vi "Worker List UI.vi"() -> ()   [LabVIEW 2020, in "FlexBlocks.lvlib"]
uses:
  FlexBlocks.lvlib
  UI State.ctl
panel:
  out "Icon":picture
  in  "New Variant":bool
  in  "Enable Variants":bool
  in  "Open Worker":bool
  in  "Values":string(tree)
  in  "New Worker":bool
  in  "Variant":i32(listbox)
  in  "Worker Search":string
  in  "Clear Search":bool
  out "Worker Name":string
  in  "Workers":i32(listbox)
  # "No variants for the selected worker"
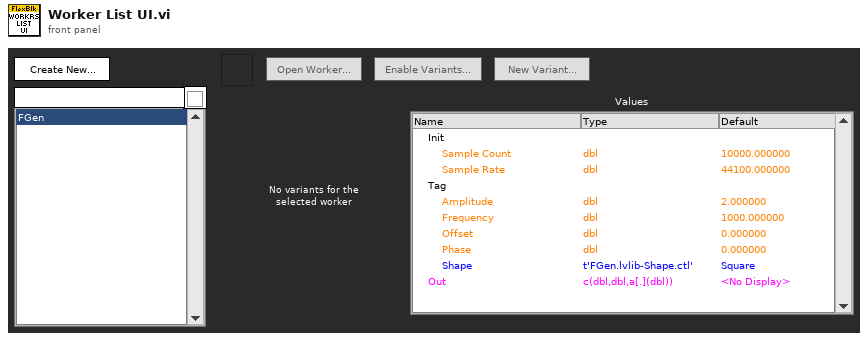
[diagram p1: front panel]
types:
  T1 = typedef "FlexBlocks.lvlib/UI State.ctl" = enum16{"Init", "Load", "Ready", "Run", "Close"}
  T2 = enum32{"Invalid", "Standard", "Closed", "Hidden", "Minimized", "Maximized"}
  T3 = enum8{"Enabled", "Disabled", "Disabled and Grayed Out"}
  T4 = typedef "imagedata.ctl" = cluster{"image type":i32, "image depth":i32, "image":u8[], "mask":u8[], "colors":u32[], "Rectangle":cluster{"left":i16, "top":i16, "right":i16, "bottom":i16}}
  T5 = typedef "FlexBlocks.lvlib/Special Terminal Indices.ctl" = cluster{"Action":i32, "Init":i32, "Tag":i32, "State in":i32, "State out":i32, "Error":i32}
  T6 = typedef "FlexBlocks.lvlib/Type Descriptor.ctl" = cluster{"Name":string, "Direction":T7, "Default":variant, "Min":variant, "Max":variant, "Step":variant, "Value Mode":T8, "Required":bool, "Connpane Index":i32, "Special Terminal":T9, "Color":u32, "Channel Path":path, "Options":string[], "Type String":string, "Sort":i32}
  T7 = typedef "FlexBlocks.lvlib/Terminal Direction.ctl" = enum16{"Sink", "Source"}
  T8 = typedef "FlexBlocks.lvlib/Value Mode.ctl" = enum16{"Normal", "Range", "Select"}
  T9 = typedef "FlexBlocks.lvlib/Special Terminal.ctl" = enum16{"None", "Action", "Init", "Tag", "State in", "State out", "Error"}
  T10 = typedef "eventvkey.ctl" = enum16{"ASCII", "Enter", "Return", "Shift", "Ctrl", "Alt", "Cmd", "Opt", "Caps", "NumLock", "Clear", "Break", "Up", "Down", "Left", "Right", "Insert", "Delete", "Home", "End", "PageUp", "PageDown", "Escape", "Help", "Pause", "ScrollLock", "F1", "F2", "F3", "F4", "F5", "F6", "F7", "F8", "F9", "F10", "F11", "F12", "F13", "F14", "F15", "F16", "F17", "F18", "F19", "F20", "F21", "F22", "F23", "F24", "Play", "VolumeUp", "VolumeDown", "Mute", "Two Byte Char"}
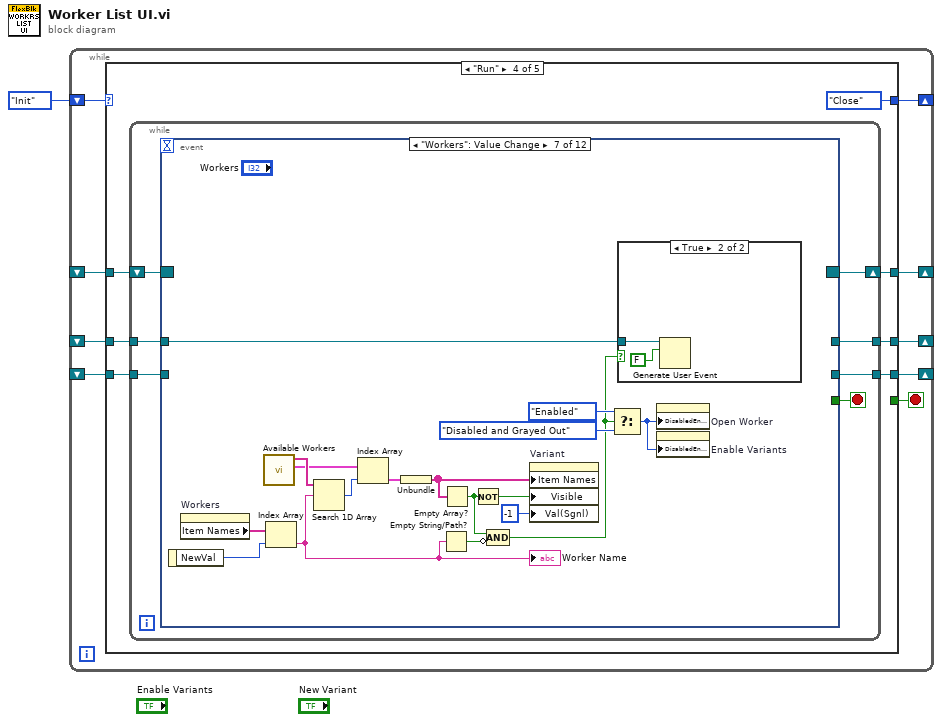
[diagram p0: block diagram]
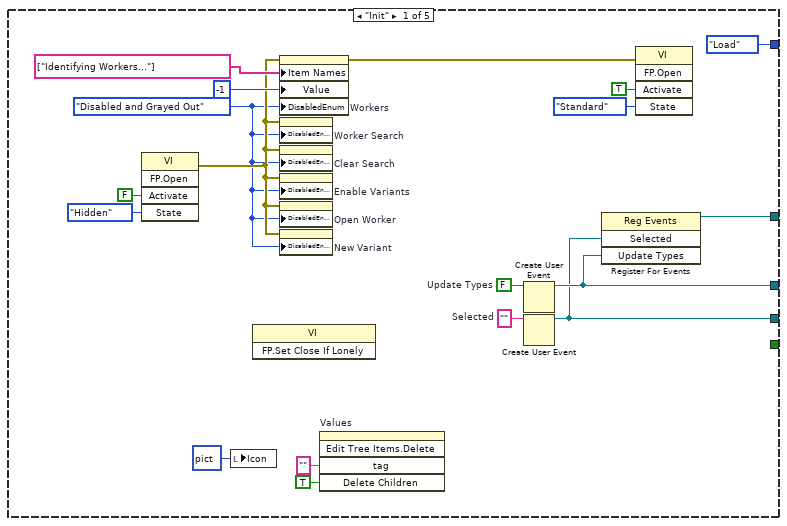
[diagram p2: hidden frame]
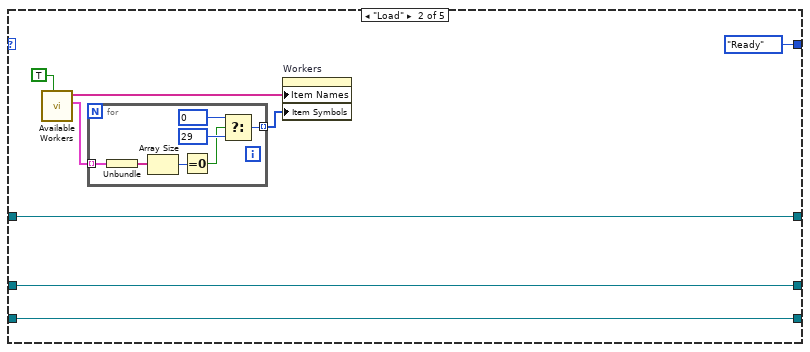
[diagram p3: hidden frame]
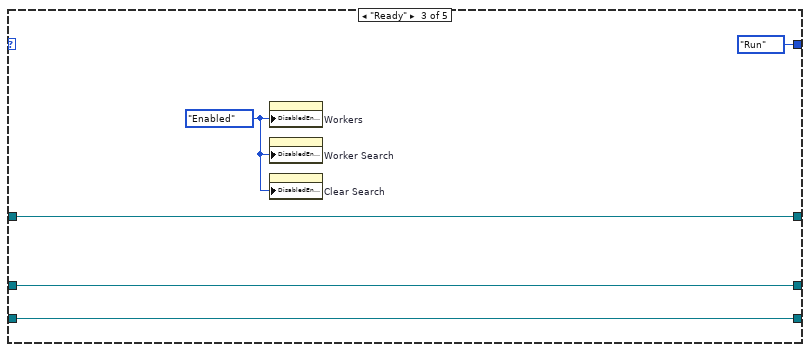
[diagram p4: hidden frame]
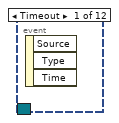
[diagram p5: hidden frame]
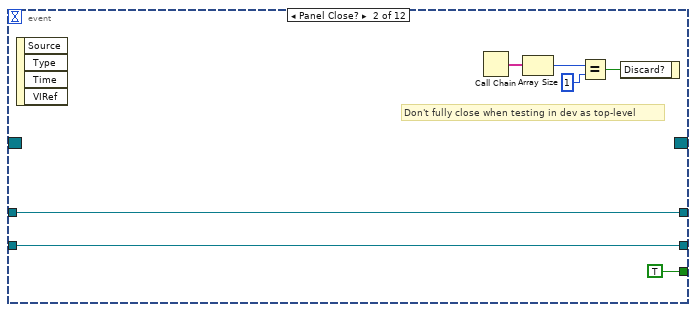
[diagram p6: hidden frame]
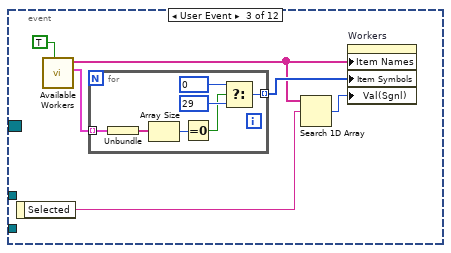
[diagram p7: hidden frame]
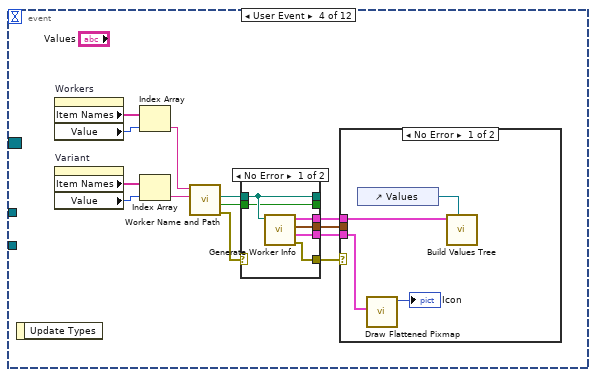
[diagram p8: hidden frame]
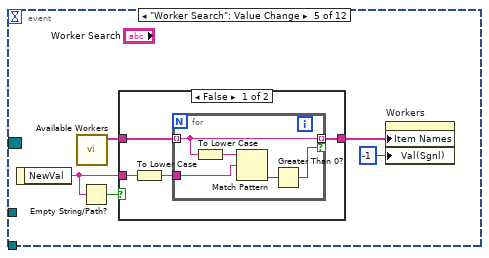
[diagram p11: hidden frame]
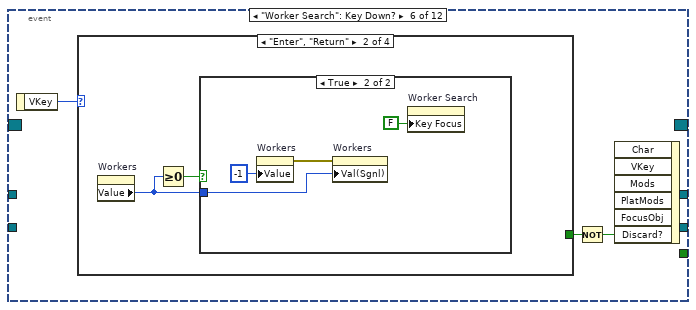
[diagram p13: hidden frame]
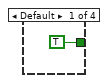
[diagram p14: hidden frame]
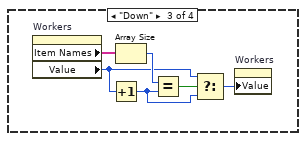
[diagram p16: hidden frame]
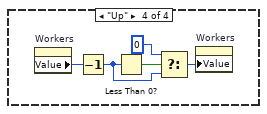
[diagram p17: hidden frame]
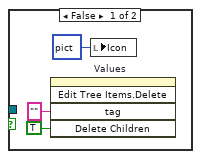
[diagram p18: hidden frame]
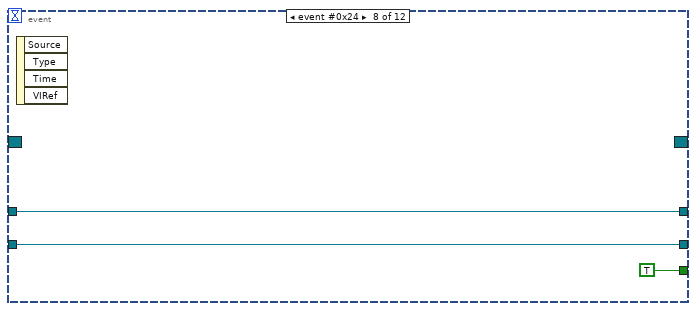
[diagram p19: hidden frame]
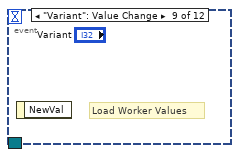
[diagram p20: hidden frame]
diagram:
  n1 = while {
    shift-right: [w9] -> _
    shift-left: UI_State."Init" ("UI State") -> [w10]
    shift-right: [w7] -> _
    shift-left: _ -> [w5]
    shift-right: [w6] -> _
    shift-left: _ -> [w4]
    shift-right: [w3] -> _
    shift-left: _ -> [w2]
    stop <- w8 stop-if-true
    n2 = case shown="\"Run\"" w10 {
      selector: w10 -> [_ _ _ _ w200]
      tunnel: [UI_State."Load" ("UI State") UI_State."Ready" ("UI State") UI_State."Run" ("UI State") UI_State."Close" ("UI State") w200] -> w9
      tunnel: [_ _ _ _ TRUE] -> w8
      tunnel: [w21 w31 w46 w52 refnum<event-registration> refnum ("Event Registration Refnum")] -> w7
      tunnel: [w14 w30 w45 w51 refnum<user-event> refnum ("Selected")] -> w6
      tunnel: w5 -> [_ w31 w46 w54 w197]
      tunnel: w4 -> [_ w30 w45 w53 w198]
      tunnel: [w15 w29 w44 w49 refnum<user-event> refnum ("Update Types")] -> w3
      tunnel: w2 -> [_ w29 w44 w50 w194]
      frame "Init" {
        w16 = FALSE  # Update Types
        w20 = ""  # Selected
        w18 = T3."Disabled and Grayed Out" ("Disabled")
        n3 = invoke class="VI" method="FP.Open"("Activate"=FALSE ("Activate?"), "State"=T2."Hidden") -> (error out=w19:errorcluster)  [unwired: 3 in, 4 out]
        n4 = local write "Icon"(picture data[5B] ("empty picture")) -> ()
        n5 = invoke class="VI" method="FP.Set Close If Lonely"() -> ()  [unwired: 3 in, 3 out]
        n6 = property on="Workers" class="LstBox (strict)"(error in=w19, "Item Names"=string[] ["Identifying Workers..."], "Value"=-1 ("Workers"), "DisabledEnum"=w18) -> (error out=w17:errorcluster)  [unwired: 1 in, 1 out]
        n7 = property on="Worker Search" class="Str"(error in=w19, "DisabledEnum"=w18) -> ()  [unwired: 1 in, 2 out]
        n8 = property on="Clear Search" class="Bool"(error in=w19, "DisabledEnum"=w18) -> ()  [unwired: 1 in, 2 out]
        n9 = property on="Enable Variants" class="Bool"(error in=w19, "DisabledEnum"=w18) -> ()  [unwired: 1 in, 2 out]
        n10 = property on="Open Worker" class="Bool"(error in=w19, "DisabledEnum"=w18) -> ()  [unwired: 1 in, 2 out]
        n11 = property on="New Variant" class="Bool"(error in=w19, "DisabledEnum"=w18) -> ()  [unwired: 1 in, 2 out]
        n12 = invoke on="Values" class="Tree (strict)" method="Edit Tree Items.Delete"("tag"="" ("Tag"), "Delete Children"=TRUE ("Delete Children?")) -> ()  [unwired: 3 in, 5 out]
        n13 = Create User Event(user event datatype=w16) -> (user event=w15:refnum<user-event>)  [unwired: 1 in, 1 out]
        n14 = Create User Event(user event datatype=w20) -> (user event=w14:refnum<user-event>)  [unwired: 1 in, 1 out]
        n15 = register-events(w14, w15) -> (reference out=w21:refnum<event-registration>)  [unwired: 2 in, 1 out]
        n16 = invoke class="VI" method="FP.Open"(error in=w17, "Activate"=TRUE ("Activate?"), "State"=T2."Standard") -> ()  [unwired: 2 in, 5 out]
      }
      frame "Load" {
        n17 = call "Available Workers.vi"("Refresh? (F)"=TRUE) -> ("Variants"=w33:cluster{"Variants":string[]}[], "Available Workers"=w34:string[])  [unwired: 9 in]
        n18 = for {
          tunnel: w33 -> [w41] mode=indexing
          tunnel: [w37] -> w32 mode=indexing
          n19 = Unbundle(w41) -> ("Variants"=w40:string[])
          n20 = Array Size(array=w40) -> (size(s)=w39:i32)
          n21 = Equal To 0?(x=w39) -> (x = 0?=w38:bool)
          n22 = Select(t=0, s=w38, f=29) -> (s? t:f=w37:i32)
        }
        n23 = property on="Workers" class="LstBox (strict)"("Item Names"=w34, "Item Symbols"=w32) -> ()  [unwired: 2 in, 2 out]
      }
      frame "Ready" {
        w47 = T3."Enabled" ("Disabled")
        n24 = property on="Workers" class="LstBox (strict)"("DisabledEnum"=w47) -> ()  [unwired: 2 in, 2 out]
        n25 = property on="Worker Search" class="Str"("DisabledEnum"=w47) -> ()  [unwired: 2 in, 2 out]
        n26 = property on="Clear Search" class="Bool"("DisabledEnum"=w47) -> ()  [unwired: 2 in, 2 out]
      }
      frame "Run" {
        n27 = while {
          shift-right: [w59] -> w52
          shift-left: w54 -> [w61]
          tunnel: w53 -> [w60]
          tunnel: [w58] -> w51
          tunnel: w50 -> [w57]
          tunnel: [w56] -> w49
          stop <- w62 stop-if-true
          n28 = event shown="[6] \"Workers\": Value Change" {
            selector: w61 -> [_ _ _ _ _ _ _ _ _ _ _ _]
            dyn-events: [_ _ _ _ _ _ _ _ _ _ _ _] -> w59
            timeout: _ -> [_ _ _ _ _ _ _ _ _ _ _ _]
            tunnel: [_ TRUE _ _ _ _ _ TRUE _ _ _ _] -> w62
            tunnel: w60 -> [_ w68 _ _ _ _ _ w167 _ _ w169 _]
            tunnel: [_ w68 _ _ _ _ _ w167 _ _ _ _] -> w58
            tunnel: w57 -> [_ w63 _ _ _ _ w144 w165 _ _ _ _]
            tunnel: [_ w63 _ _ _ _ _ w165 _ _ _ _] -> w56
            event Timeout {
              n29 = event-data() -> ()  [unwired: 1 in, 3 out]
            }
            event Panel Close? {
              # "Don't fully close when testing in dev as top-level"
              n30 = event-data() -> ()  [unwired: 1 in, 4 out]
              n31 = Call Chain() -> (call chain=w67:string[])
              n32 = Array Size(array=w67) -> (size(s)=w66:i32)
              n33 = Equal?(x=w66, y=1) -> (x = y?=w64:bool)
              n34 = event-data("Discard?"=w64) -> ()  [unwired: 1 in, 1 out]
            }
            event User Event {
              n35 = event-data() -> ("Selected"=w71:string)  [unwired: 1 in]
              n36 = call "Available Workers.vi"("Refresh? (F)"=TRUE) -> ("Variants"=w74:cluster{"Variants":string[]}[], "Available Workers"=w72:string[])  [unwired: 9 in]
              n37 = for {
                tunnel: w74 -> [w80] mode=indexing
                tunnel: [w76] -> w73 mode=indexing
                n38 = Unbundle(w80) -> ("Variants"=w79:string[])
                n39 = Array Size(array=w79) -> (size(s)=w78:i32)
                n40 = Equal To 0?(x=w78) -> (x = 0?=w77:bool)
                n41 = Select(t=0, s=w77, f=29) -> (s? t:f=w76:i32)
              }
              n42 = Search 1D Array(1D array=w72, element=w71) -> (index of element=w70:i32)  [unwired: 1 in]
              n43 = property on="Workers" class="LstBox (strict)"("Item Names"=w72, "Item Symbols"=w73, "Val(Sgnl)"=w70) -> ()  [unwired: 2 in, 2 out]
            }
            event User Event {
              n44 = event-data() -> ()  [unwired: 1 in, 1 out]
              n45 = property on="Workers" class="LstBox (strict)"() -> ("Item Names"=w92:string[], "Value"=w91:i32)  [unwired: 2 in, 2 out]
              n46 = property on="Variant" class="LstBox (strict)"() -> ("Item Names"=w89:string[], "Value"=w90:i32)  [unwired: 2 in, 2 out]
              n47 = Index Array(array=w92, index=w91) -> (element=w87:string)
              n48 = Index Array(array=w89, index=w90) -> (element=w88:string)
              n49 = call "Worker Name and Path.vi"("Variant"=w88, "Worker"=w87) -> ("error out"=w94:errorcluster, "Is Worker Variant"=w93:bool, "lvlib Path"=w95:path)  [unwired: 6 in, 1 out]
              n50 = case shown="No Error" w94 {
                selector: w94 -> [_ w106]
                tunnel: [w105 w106] -> w86
                tunnel: [w104 _] -> w85
                tunnel: [w103 _] -> w84
                tunnel: [w102 _] -> w83
                tunnel: w95 -> [w101 _]
                tunnel: [w101 _] -> _
                tunnel: w93 -> [w100 _]
                tunnel: [w100 _] -> _
                frame No Error {
                  n51 = call "Generate Worker Info.vi"("Worker lvlib"=w101) -> ("error out"=w105:errorcluster, "Icon"=w104:T4, "Special Terminals"=w103:T5, "Type Descriptors"=w102:T6[])  [unwired: 7 in]
                }
                frame Error {
                }
              }
              n52 = case shown="No Error" w86 {
                tunnel: w85 -> [w99 _]
                tunnel: w84 -> [_ _]
                tunnel: w83 -> [w97 _]
                frame No Error {
                  n53 = control-ref of="Values"() -> (w96:refnum<vi>)
                  n54 = call <vilib>:"Draw Flattened Pixmap.vi"("image data"=w99) -> ("new picture"=→"Icon":picture)  [unwired: 8 in]
                  n55 = call "Build Values Tree.vi"("Tree"=w96, "Types"=w97) -> ()  [unwired: 10 in]
                }
                frame Error {
                }
              }
            }
            event "Worker Search": Value Change {
              n56 = event-data() -> ("NewVal"=w110:string)  [unwired: 1 in]
              n57 = call "Available Workers.vi"() -> ("Available Workers"=w111:string[])  [unwired: 10 in, 1 out]
              n58 = Empty String/Path?(string/path=w110) -> (empty?=w109:bool)
              n59 = case shown="False" w109 {
                tunnel: w111 -> [w115 w121]
                tunnel: w110 -> [w114 _]
                tunnel: [w113 w121] -> w108
                frame False {
                  n60 = To Lower Case(string=w114) -> (all lower case string=w112:string)
                  n61 = for {
                    tunnel: w115 -> [w120] mode=indexing
                    tunnel: w112 -> [w119]
                    tunnel: [w120] -> w113 mode=indexing if=w117
                    n62 = To Lower Case(string=w120) -> (all lower case string=w116:string)
                    n63 = Match Pattern(string=w116, regular expression=w119) -> (offset past match=w118:i32)  [unwired: 1 in, 3 out]
                    n64 = Greater Than 0?(x=w118) -> (x > 0?=w117:bool)
                  }
                }
                frame True {
                }
              }
              n65 = property on="Workers" class="LstBox (strict)"("Item Names"=w108, "Val(Sgnl)"=-1 ("Workers")) -> ()  [unwired: 2 in, 2 out]
            }
            event "Worker Search": Key Down? {
              n66 = event-data() -> ("VKey"=w124:T10)  [unwired: 1 in]
              n67 = case shown="\"Enter\", \"Return\"" w124 {
                tunnel: [TRUE _ _ _] -> w123
                frame Default {
                }
                frame "Enter", "Return" {
                  n68 = property on="Workers" class="LstBox (strict)"() -> ("Value"=w126:i32)  [unwired: 2 in, 2 out]
                  n69 = Greater Or Equal To 0?(x=w126) -> (x >= 0?=w127:bool)
                  n70 = case shown="True" w127 {
                    tunnel: w126 -> [_ w129]
                    frame False {
                    }
                    frame True {
                      n71 = property on="Workers" class="LstBox (strict)"("Value"=-1 ("Workers")) -> (error out=w128:errorcluster)  [unwired: 2 in, 1 out]
                      n72 = property on="Workers" class="LstBox (strict)"(error in=w128, "Val(Sgnl)"=w129) -> ()  [unwired: 1 in, 2 out]
                      n73 = property on="Worker Search" class="Str"("Key Focus"=FALSE) -> ()  [unwired: 2 in, 2 out]
                    }
                  }
                }
                frame "Down" {
                  n74 = property on="Workers" class="LstBox (strict)"() -> ("Item Names"=w137:string[], "Value"=w134:i32)  [unwired: 2 in, 2 out]
                  n75 = Increment(x=w134) -> (x+1=w132:i32)
                  n76 = Array Size(array=w137) -> (size(s)=w136:i32)
                  n77 = Equal?(x=w136, y=w132) -> (x = y?=w135:bool)
                  n78 = Select(t=w134, s=w135, f=w132) -> (s? t:f=w133:i32)
                  n79 = property on="Workers" class="LstBox (strict)"("Value"=w133) -> ()  [unwired: 2 in, 2 out]
                }
                frame "Up" {
                  n80 = property on="Workers" class="LstBox (strict)"() -> ("Value"=w142:i32)  [unwired: 2 in, 2 out]
                  n81 = Decrement(x=w142) -> (x-1=w140:i32)
                  n82 = Less Than 0?(x=w140) -> (x < 0?=w141:bool)
                  n83 = Select(t=0, s=w141, f=w140) -> (s? t:f=w138:i32)
                  n84 = property on="Workers" class="LstBox (strict)"("Value"=w138) -> ()  [unwired: 2 in, 2 out]
                }
              }
              n85 = Not(x=w123) -> (.not. x?=w122:bool)
              n86 = event-data("Discard?"=w122) -> ()  [unwired: 6 in, 1 out]
            }
            event "Workers": Value Change {
              n87 = event-data() -> ("NewVal"=w158:i32)  [unwired: 1 in]
              n88 = property on="Workers" class="LstBox (strict)"() -> ("Item Names"=w159:string[])  [unwired: 2 in, 2 out]
              n89 = call "Available Workers.vi"() -> ("Variants"=w156:cluster{"Variants":string[]}[], "Available Workers"=w157:string[])  [unwired: 10 in]
              n90 = Index Array(array=w159, index=w158) -> (element=w151:string)
              "Worker Name" <- w151
              n91 = Search 1D Array(1D array=w157, element=w151) -> (index of element=w155:i32)  [unwired: 1 in]
              n92 = Index Array(array=w156, index=w155) -> (element=w154:cluster{"Variants":string[]})
              n93 = Unbundle(w154) -> ("Variants"=w153:string[])
              n94 = Empty String/Path?(string/path=w151) -> (empty?=w150:bool)
              n95 = Empty Array?(array=w153) -> (empty?=w148:bool)
              n96 = Not(x=w148) -> (.not. x?=w149:bool)
              n97 = Compound Arithmetic op=AND(w148, invert w150) -> (w143:bool)
              n98 = property on="Variant" class="LstBox (strict)"("Item Names"=w153, "Visible"=w149, "Val(Sgnl)"=-1 ("Value (Signaling)")) -> ()  [unwired: 2 in, 2 out]
              n99 = Select(t=T3."Enabled" ("Disabled"), s=w143, f=T3."Disabled and Grayed Out" ("Disabled")) -> (s? t:f=w145:T3)
              n100 = case shown="True" w143 {
                tunnel: w144 -> [_ w164]
                frame False {
                  n101 = invoke on="Values" class="Tree (strict)" method="Edit Tree Items.Delete"("tag"="" ("Tag"), "Delete Children"=TRUE ("Delete Children?")) -> ()  [unwired: 3 in, 5 out]
                  n102 = local write "Icon"(picture data[5B] ("empty picture")) -> ()
                }
                frame True {
                  n103 = Generate User Event(user event=w164, event data cluster=FALSE ("event data")) -> ()  [unwired: 2 in, 2 out]
                }
              }
              n104 = property on="Open Worker" class="Bool"("DisabledEnum"=w145) -> ()  [unwired: 2 in, 2 out]
              n105 = property on="Enable Variants" class="Bool"("DisabledEnum"=w145) -> ()  [unwired: 2 in, 2 out]
            }
            event event #0x24 {
              n106 = event-data() -> ()  [unwired: 1 in, 4 out]
            }
            event "Variant": Value Change {
              # "Load Worker Values"
              n107 = event-data() -> ()  [unwired: 1 in, 1 out]
            }
            event "Clear Search": Value Change {
              n108 = event-data() -> ()  [unwired: 1 in, 6 out]
              n109 = property on="Worker Search" class="Str"("Val(Sgnl)"="" ("Value (Signaling)")) -> ()  [unwired: 2 in, 2 out]
            }
            event "New Worker": Value Change {
              n110 = event-data() -> ()  [unwired: 1 in, 1 out]
              n111 = call "New Worker Name UI.vi"() -> ("New Project?"=w170:bool, "Add to Project"=w171:refnum<vi>, "Cancelled?"=w173:bool, "New Name"=w172:string)  [unwired: 8 in]
              n112 = case shown="False" w173 {
                tunnel: w172 -> [w174 _]
                tunnel: w171 -> [w178 _]
                tunnel: w170 -> [w177 _]
                tunnel: w169 -> [w175 _]
                frame False {
                  n113 = call "Make New Worker.vi"("New Project?"=w177, "Add to Project (None)"=w178, "New Worker Name"=w174) -> ("error out"=w176:errorcluster)  [unwired: 8 in]
                  n114 = case shown="No Error" w176 {
                    selector: w176 -> [_ w181]
                    tunnel: w175 -> [w180 _]
                    tunnel: w174 -> [w179 _]
                    frame No Error {
                      n115 = Generate User Event(user event=w180, event data cluster=w179) -> ()  [unwired: 2 in, 2 out]
                    }
                    frame Error {
                      n116 = call <vilib>:"Simple Error Handler.vi"("error in (no error)"=w181) -> ()  [unwired: 4 in, 5 out]
                    }
                  }
                }
                frame True {
                }
              }
            }
            event "Open Worker": Value Change; "Workers", "Variant": Double Click {
              n117 = event-data() -> ()  [unwired: 1 in, 1 out]
              n118 = property on="Open Worker" class="Bool"() -> ("DisabledEnum"=w184:T3)  [unwired: 2 in, 2 out]
              n119 = Equal?(x=w184, y=T3."Enabled") -> (x = y?=w182:bool)
              n120 = case shown="True" w182 {
                frame False {
                }
                frame True {
                  n121 = property on="Workers" class="LstBox (strict)"() -> ("Item Names"=w192:string[], "Value"=w191:i32)  [unwired: 2 in, 2 out]
                  n122 = property on="Variant" class="LstBox (strict)"() -> ("Item Names"=w188:string[], "Value"=w189:i32)  [unwired: 2 in, 2 out]
                  n123 = Index Array(array=w192, index=w191) -> (element=w190:string)
                  n124 = Index Array(array=w188, index=w189) -> (element=w187:string)
                  n125 = call "Worker Name and Path.vi"("Variant"=w187, "Worker"=w190) -> ("lvlib Path"=w186:path)  [unwired: 6 in, 3 out]
                  n126 = invoke class="App" method="Open.LV Document"("path"=w186, "Interactive?"=FALSE) -> ()  [unwired: 3 in, 5 out]
                }
              }
            }
          }
        }
      }
      frame "Close" {
        n127 = Unregister For Events(event registration refnum=w197) -> ()  [unwired: 1 in, 1 out]
        n128 = Destroy User Event(user event=w194) -> ()  [unwired: 1 in, 1 out]
        n129 = Destroy User Event(user event=w198) -> ()  [unwired: 1 in, 1 out]
      }
    }
  }
